vi "tic tac toe.vi"() -> ()   [LabVIEW 2017]
uses:
  <vilib>/event_ctls.llb/eventvkey.ctl
  <vilib>/DAQmx/write.llb/DAQmx Write (Digital Bool 1Line 1Point).vi
  <vilib>/DAQmx/read.llb/DAQmx Read (Counter U32 1Chan 1Samp).vi
  <vilib>/DAQmx/create/channels.llb/DAQmx Create Channel (CO-Pulse Generation-Frequency).vi
  <vilib>/DAQmx/configure/timing.llb/DAQmx Timing (Implicit).vi
  <vilib>/DAQmx/create/channels.llb/DAQmx Create Channel (CI-Count Edges).vi
  <vilib>/DAQmx/create/channels.llb/DAQmx Create Channel (DO-Digital Output).vi
  <vilib>/DAQmx/miscellaneous.llb/DAQmx Fill In Error Info.vi
  <resource>/objmgr/daqmx.rc
  <vilib>/Analysis/NI_AALBase.lvlib
panel:
  in  "btn pause":bool
  out "Станд. отклонение O":dbl format="%0.2f"
  out "Станд. отклонение X":dbl format="%0.2f"
  out "Мат. ождание O":dbl
  out "Мат. ождание X":dbl
  out "Гистограмма ходов O":T1(graph)
  out "Гистограмма ходов X":T1(graph)
  out "ВРЕМЯ ПОСЛЕДНЕГО ХОДА (сек.)":dbl
  out "Массив времён O":dbl[](array[numeric])
  out "Массив времён X":dbl[](array[numeric])
  out "Результат":string
  in  "btn new game":bool
  out "Boolean":bool
  in  "Игровое поле":i32[][](array[ring]) items=["", "X", "0"]
  out "ХОД":string
  in  "btn stop":bool
  # "\"Крестики-нолики 15x15\""
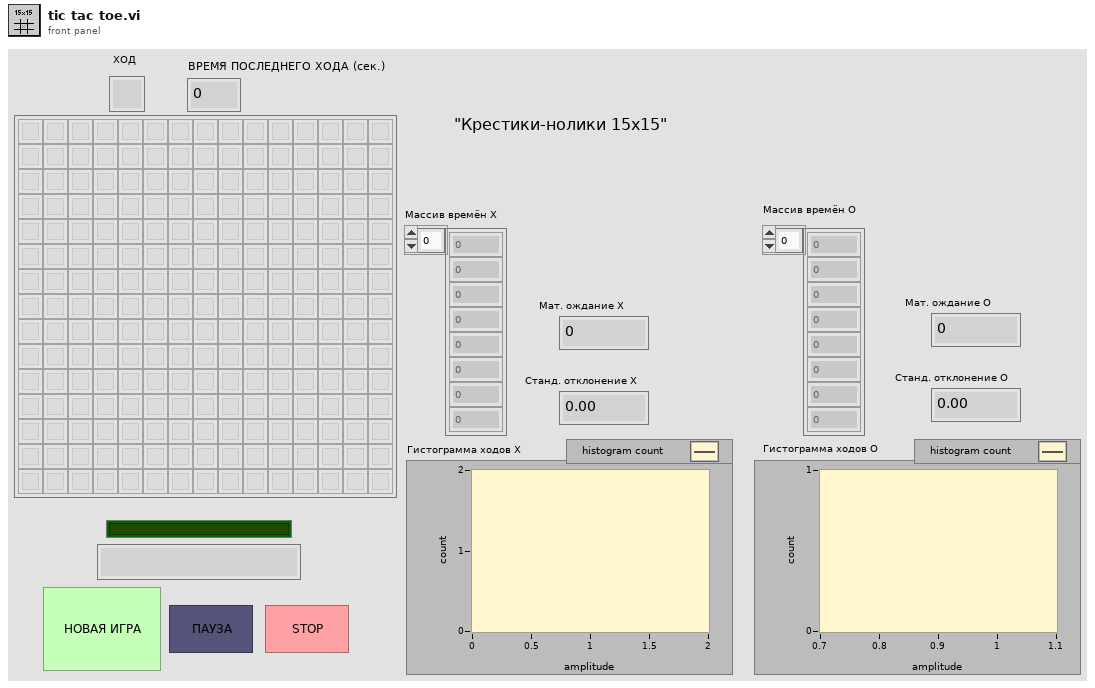
[diagram p1: front panel]
types:
  T1 = cluster{"X Values":dbl[], "Histogram: h(x)":i32[]}
  T2 = enum8{"Enabled", "Disabled", "Disabled and Grayed Out"}
  T3 = typedef "eventvkey.ctl" = enum16{"ASCII", "Enter", "Return", "Shift", "Ctrl", "Alt", "Cmd", "Opt", "Caps", "NumLock", "Clear", "Break", "Up", "Down", "Left", "Right", "Insert", "Delete", "Home", "End", "PageUp", "PageDown", "Escape", "Help", "Pause", "ScrollLock", "F1", "F2", "F3", "F4", "F5", "F6", "F7", "F8", "F9", "F10", "F11", "F12", "F13", "F14", "F15", "F16", "F17", "F18", "F19", "F20", "F21", "F22", "F23", "F24", "Play", "VolumeUp", "VolumeDown", "Mute", "Two Byte Char"}
  T4 = typedef "LVPoint32TypeDef.ctl" = cluster{"Horizontal":i32, "Vertical":i32}
  T5 = typedef "LVPositionTypeDef.ctl" = cluster{"Left":i32, "Top":i32}
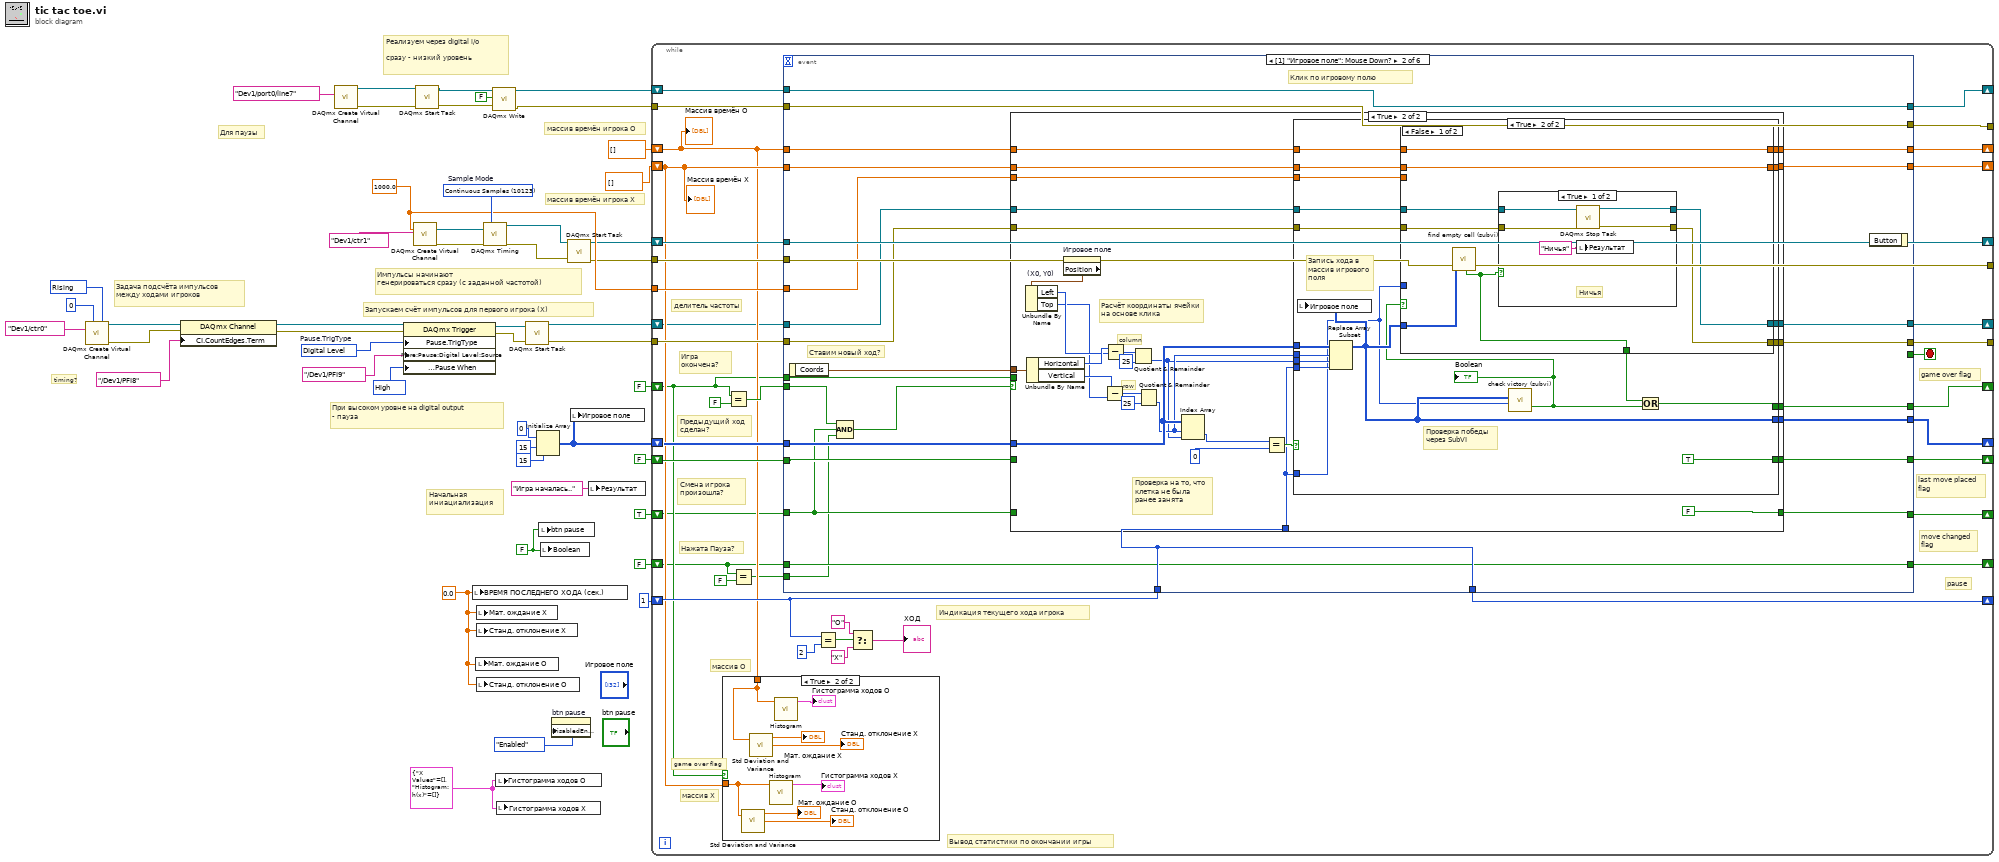
[diagram p0: block diagram]
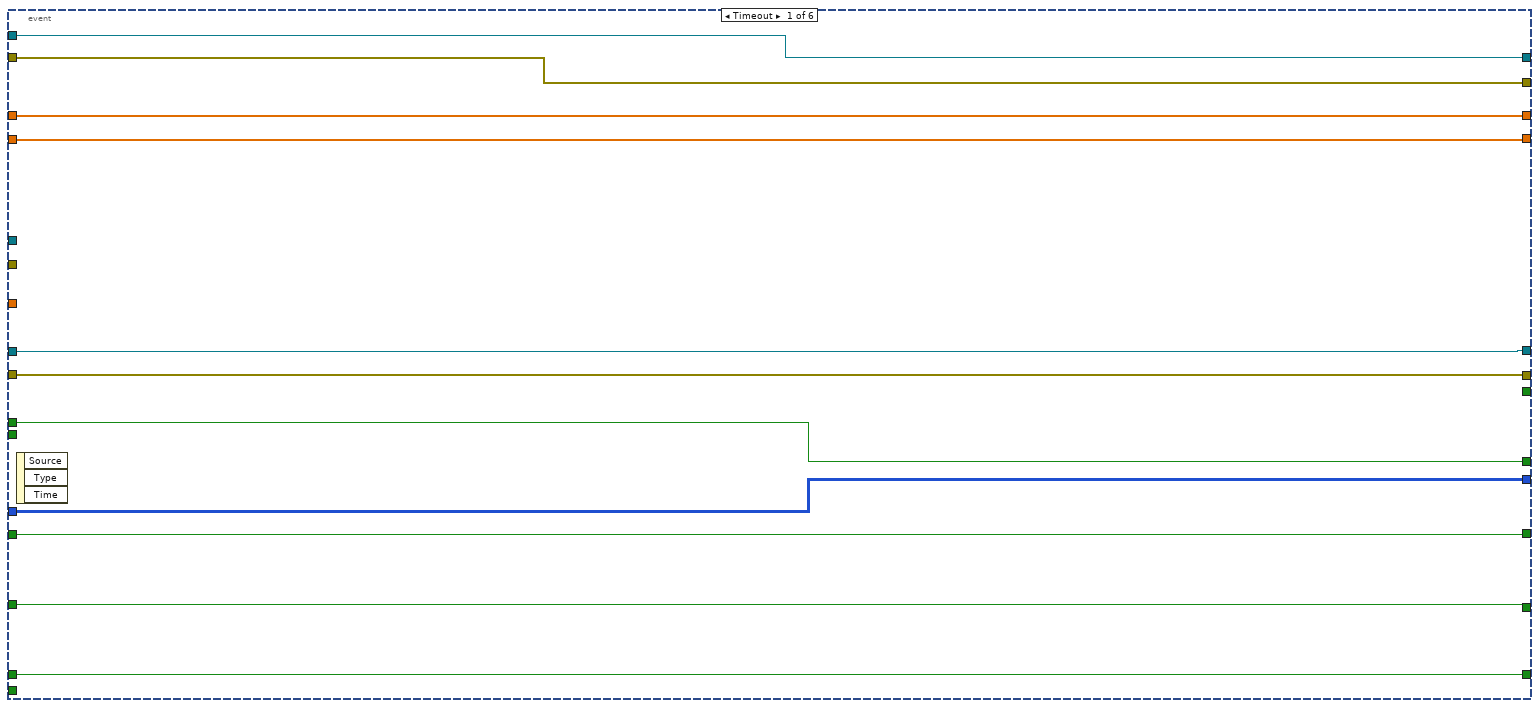
[diagram p3: hidden frame]
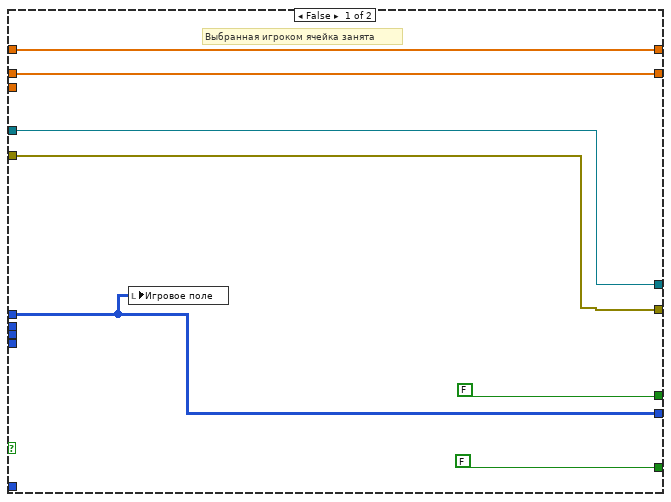
[diagram p5: hidden frame]
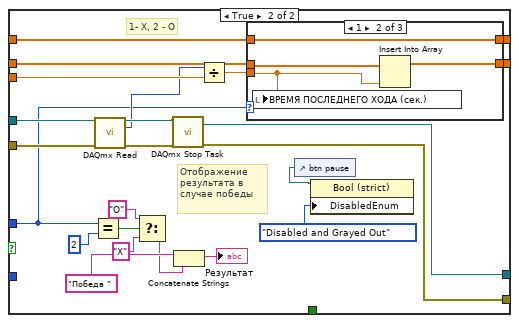
[diagram p7: hidden frame]
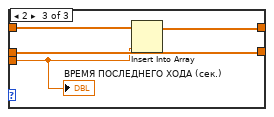
[diagram p9: hidden frame]
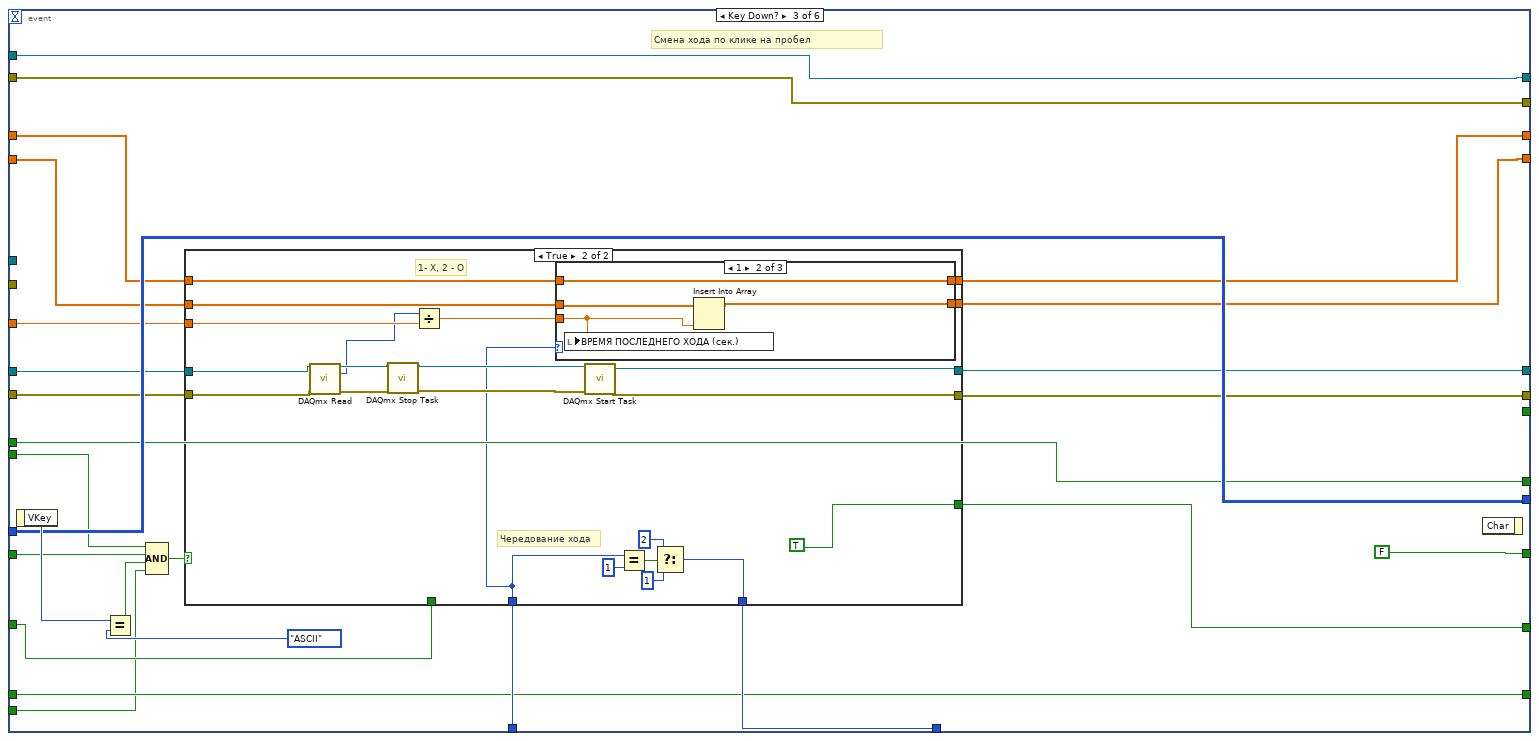
[diagram p10: hidden frame]
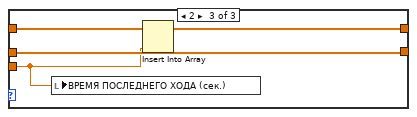
[diagram p13: hidden frame]
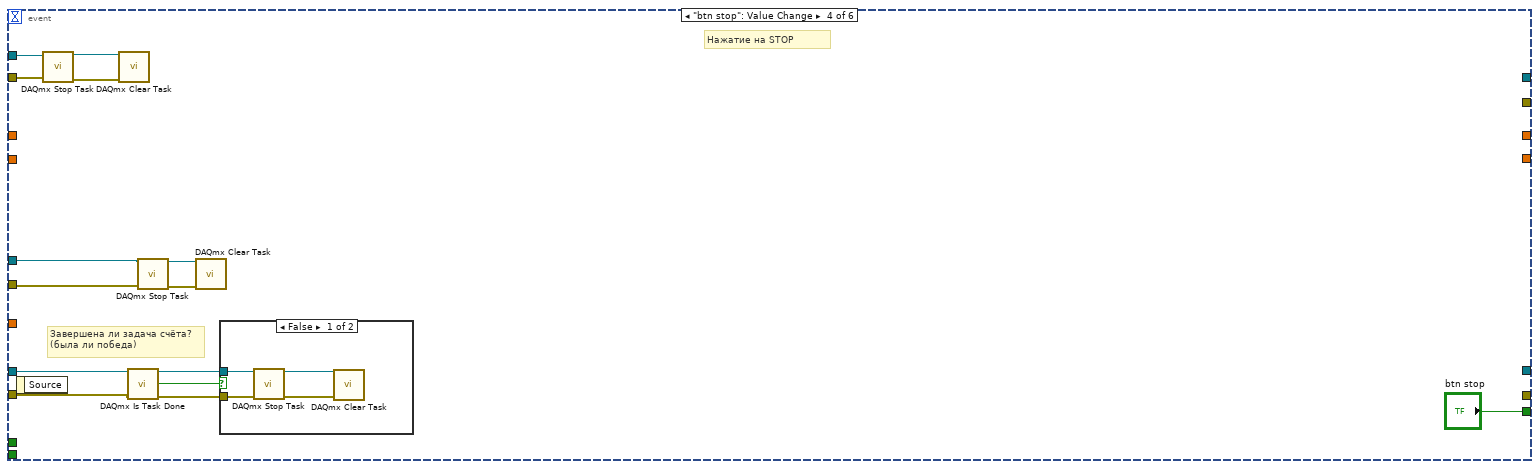
[diagram p14: hidden frame]
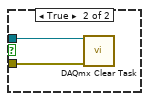
[diagram p15: hidden frame]
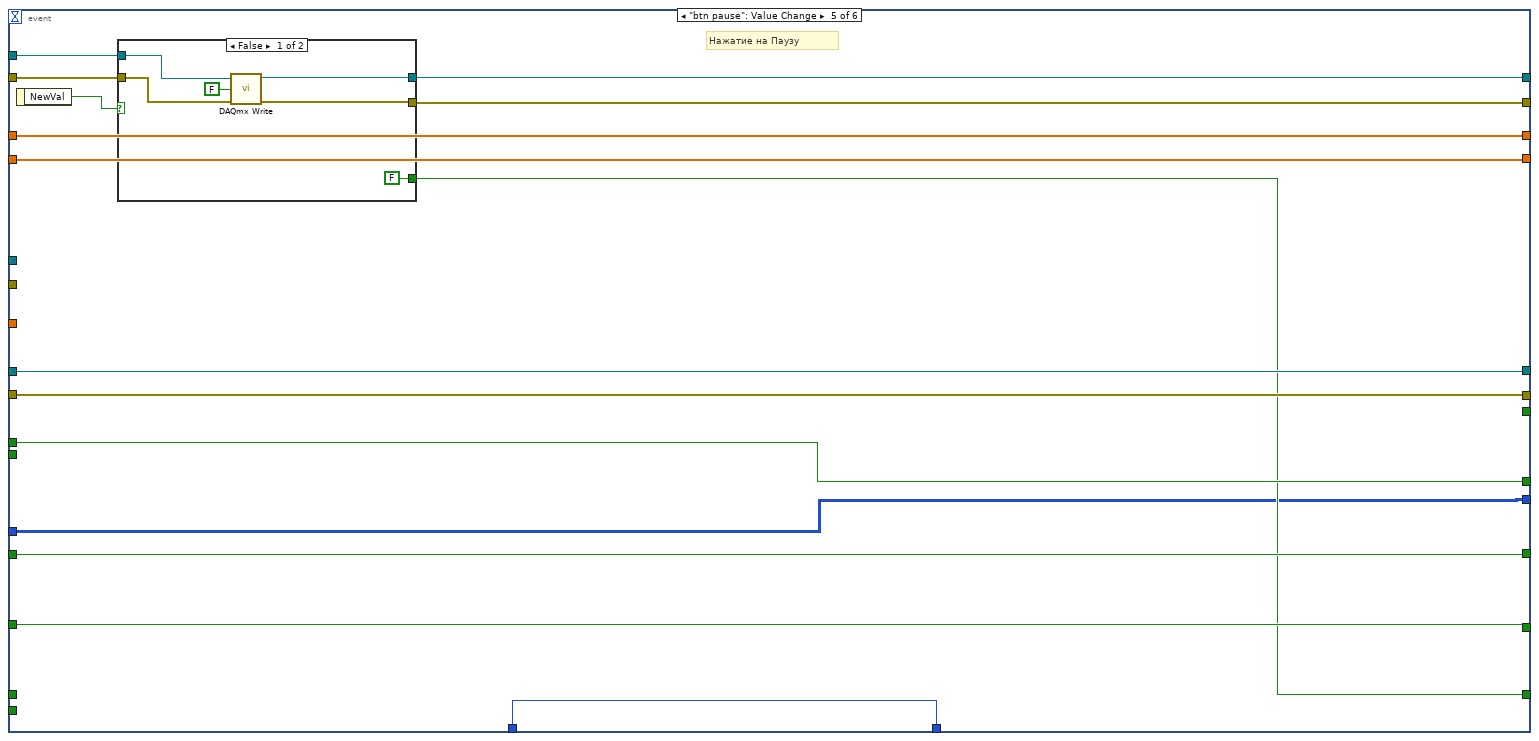
[diagram p16: hidden frame]
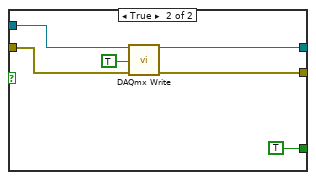
[diagram p17: hidden frame]
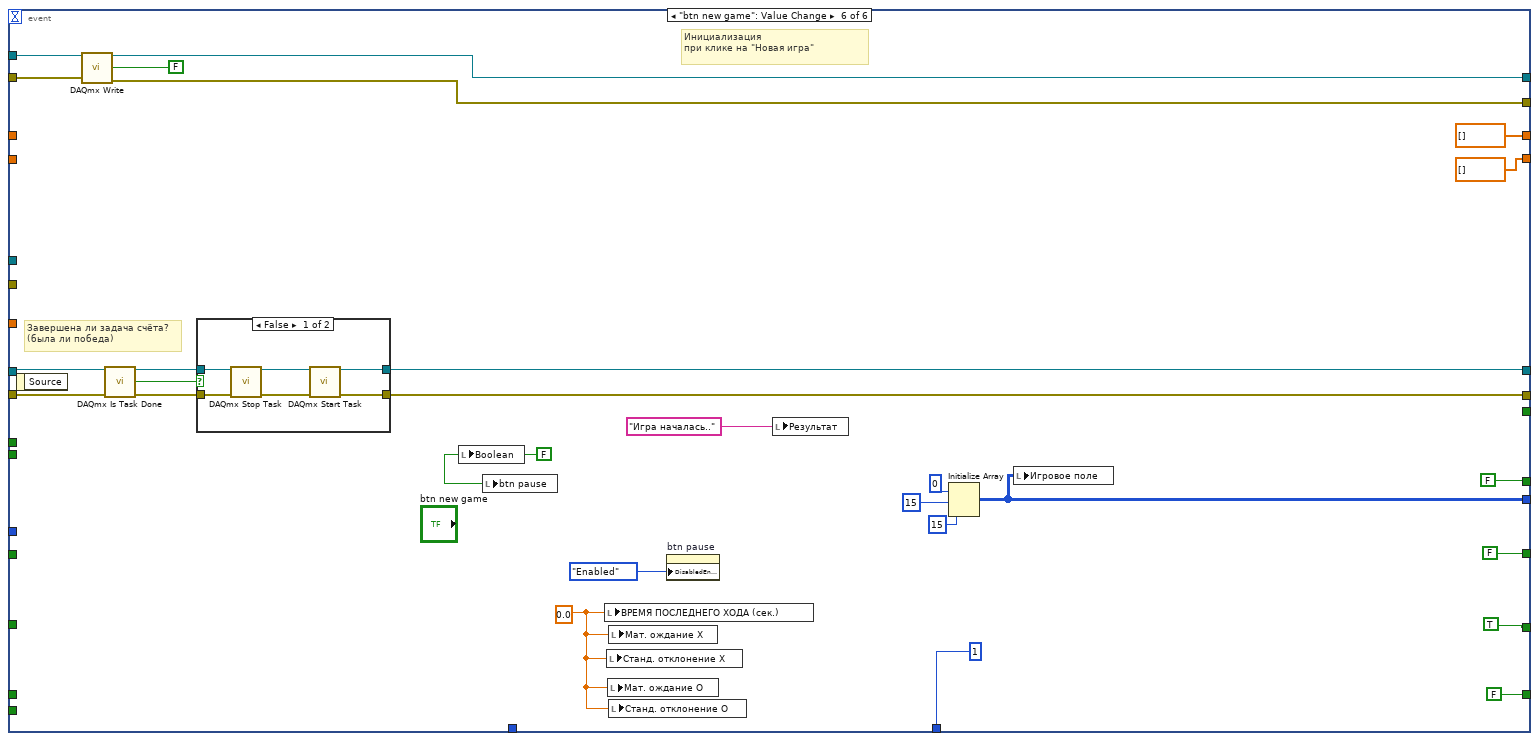
[diagram p18: hidden frame]
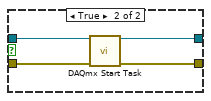
[diagram p19: hidden frame]
diagram:
  w1 = T1 {"X Values"=[], "Histogram: h(x)"=[]} ("Гистограмма ходов O")
  w2 = 0.0 ("Время последнего хода")
  w13 = 10192 items=["High"=10192, "Low"=10214] ("Pause When")
  w15 = 10152 items=["Analog Level"=10101, "Analog Window"=10103, "Digital Level"=10152, "Digital Pattern"=10398, "None"=10230]  # Pause.TrigType
  w32 = 10280 items=["Rising"=10280, "Falling"=10171] ("edge")
  w39 = 10123 items=["Finite Samples"=10178, "Continuous Samples"=10123, "Hardware Timed Single Point"=12522]  # Sample Mode
  w28 = 1000.0 ("frequency")
  w6 = FALSE
  # "При высоком уровне на digital output\n- пауза"
  # "Реализуем через digital i/o\n\nсразу - низкий уровень"
  # "Для паузы"
  # "массив времён игрока O"
  # "массив времён игрока X"
  # "Запускаем счёт импульсов для первого игрока (X)"
  # "Задача подсчёта импульсов\nмежду ходами игроков"
  # "timing?"
  # "Импульсы начинают\nгенерироваться сразу (с заданной частотой)"
  # "Начальная иниациализация"
  n1 = call-poly <vilib>:"DAQmx Create Virtual Channel.vi"("initial count"=u32 0, "edge"=w32, "counter"=tag "Dev1/ctr0") -> ("task out"=w30:refnum<k21>, "error out"=w29:errorcluster)  [unwired: 11 in]
  n2 = property class="DAQmx Channel"(reference=w30, error in=w29, "CI.CountEdges.Term"=tag "/Dev1/PFI8" ("CI.Period.Term")) -> (reference out=w10:refnum<k21>, error out=w9:errorcluster)
  n3 = call-poly <vilib>:"DAQmx Create Virtual Channel.vi"("lines"=tag "Dev1/port0/line7") -> ("task out"=w20:refnum<k21>, "error out"=w19:errorcluster)  [unwired: 13 in]
  n4 = property class="DAQmx Trigger"(reference=w10, error in=w9, "Pause.TrigType"=w15, "More:Pause:Digital Level:Source"=tag "/Dev1/PFI9" ("Pause Trigger Source"), "More:Pause:Digital Level:Pause When"=w13) -> (reference out=w12:refnum<k21>, error out=w11:errorcluster)
  n5 = call-poly <vilib>:"DAQmx Create Virtual Channel.vi"("frequency"=w28, "counter"=tag "Dev1/ctr1") -> ("task out"=w37:refnum<k21>, "error out"=w38:errorcluster)  [unwired: 12 in]
  n6 = call <vilib>:"DAQmx Start Task.vi"("task/channels in"=w20, "error in"=w19) -> ("task out"=w17:refnum<k21>, "error out"=w16:errorcluster)  [unwired: 12 in]
  n7 = local write "ВРЕМЯ ПОСЛЕДНЕГО ХОДА (сек.)"(w2) -> ()
  n8 = local write "Мат. ождание O"(w2) -> ()
  n9 = local write "Мат. ождание X"(w2) -> ()
  n10 = local write "Станд. отклонение X"(w2) -> ()
  n11 = local write "Станд. отклонение O"(w2) -> ()
  n12 = call-poly <vilib>:"DAQmx Timing.vi"("task/channels in"=w37, "sample mode"=w39, "error in"=w38) -> ("task out"=w36:refnum<k21>, "error out"=w35:errorcluster)  [unwired: 11 in]
  n13 = call-poly <vilib>:"DAQmx Write.vi"("task/channels in"=w17, "data"=FALSE, "error in"=w16) -> ("task out"=w8:refnum<k21>, "error out"=w7:errorcluster)  [unwired: 10 in, 1 out]
  n14 = local write "Гистограмма ходов O"(w1) -> ()
  n15 = local write "Гистограмма ходов X"(w1) -> ()
  n16 = call <vilib>:"DAQmx Start Task.vi"("task/channels in"=w12, "error in"=w11) -> ("task out"=w27:refnum<k21>, "error out"=w26:errorcluster)  [unwired: 12 in]
  n17 = Initialize Array(0 ("dimension size"), 15 ("dimension size"), 15 ("dimension size")) -> (w42:i32[][])
  n18 = local write "btn pause"(w6) -> ()
  n19 = local write "Boolean"(w6) -> ()
  n20 = property on="btn pause" class="Bool (strict)"("DisabledEnum"=T2."Enabled" ("Disabled")) -> ()  [unwired: 2 in, 2 out]
  n21 = call <vilib>:"DAQmx Start Task.vi"("task/channels in"=w36, "error in"=w35) -> ("task out"=w25:refnum<k21>, "error out"=w24:errorcluster)  [unwired: 12 in]
  n22 = local write "Игровое поле"(w42) -> ()
  n23 = local write "Результат"("Игра началась.." ("Результат")) -> ()
  n24 = while {
    shift-right: [w78] -> _
    shift-left: w42 -> [w79]
    shift-right: [w75] -> _
    shift-left: 1 ("f") -> [w76]
    shift-right: [w77] -> _
    shift-left: FALSE ("Победа") -> [w55]
    shift-right: [w74] -> _
    shift-left: FALSE -> [w73]
    shift-right: [w72] -> _
    shift-left: TRUE -> [w49]
    shift-right: [w69] -> _
    shift-left: w27 -> [w50]
    tunnel: w26 -> [w68]
    tunnel: w28 -> [w62]
    shift-right: [w67] -> _
    shift-left: w25 -> [w67]
    tunnel: w24 -> [w66]
    tunnel: [w66] -> _
    tunnel: [w65] -> _
    shift-right: [w64] -> _
    shift-left: dbl[] [] -> [w61]
    shift-right: [w63] -> _
    shift-left: dbl[] [] -> [w60]
    tunnel: w7 -> [w59]
    tunnel: [w58] -> _
    shift-right: [w56] -> _
    shift-left: w8 -> [w57]
    shift-right: [w54] -> _
    shift-left: FALSE -> [w52]
    stop <- w80 stop-if-true
    # "Нажата Пауза?"
    # "pause"
    # "делитель частоты"
    # "массив O"
    # "массив X"
    # "Вывод статистики по окончании игры"
    # "game over flag"
    # "Предыдущий ход сделан?"
    # "Смена игрока произошла?"
    # "Игра окончена?"
    # "move changed flag"
    # "last move placed\nflag"
    # "Индикация текущего хода игрока"
    # "game over flag"
    n25 = case shown="True" w55 {
      tunnel: w61 -> [_ w91]
      tunnel: w60 -> [_ w89]
      frame False {
      }
      frame True {
        n26 = call <vilib>:"Std Deviation and Variance.vi"("X"=w91) -> ("mean"=→"Мат. ождание O":dbl, "standard deviation"=→"Станд. отклонение O":dbl)  [unwired: 1 in, 1 out]
        n27 = call <vilib>:"Std Deviation and Variance.vi"("X"=w89) -> ("mean"=→"Мат. ождание X":dbl, "standard deviation"=→"Станд. отклонение X":dbl)  [unwired: 1 in, 1 out]
        n28 = call <vilib>:"Histogram.vi"("X"=w91) -> ("Histogram Graph"=→"Гистограмма ходов X":T1)  [unwired: 7 in, 3 out]
        n29 = call <vilib>:"Histogram.vi"("X"=w89) -> ("Histogram Graph"=→"Гистограмма ходов O":T1)  [unwired: 7 in, 3 out]
      }
    }
    n30 = Equal?(x=w55, y=FALSE) -> (x = y?=w70:bool)
    n31 = Equal?(x=w52, y=FALSE) -> (x = y?=w51:bool)
    n32 = event shown="[1] \"Игровое поле\": Mouse Down?" {
      selector: _ -> [_ _ _ _ _ _]
      dyn-events: _ -> [_ _ _ _ _ _]
      timeout: _ -> [_ _ _ _ _ _]
      tunnel: w79 -> [w94 w128 w263 _ w329 _]
      tunnel: w76 -> [_ w124 w266 _ w326 _]
      tunnel: [_ _ _ "btn stop" _ _] -> w80
      tunnel: [w94 w126 w263 _ w329 w376] -> w78
      tunnel: [w98 w127 w251 _ w333 FALSE] -> w77
      tunnel: w70 -> [_ w108 w246 _ _ _]
      tunnel: [_ w124 w265 _ w326 1] -> w75
      tunnel: [w102 w125 FALSE _ w335 FALSE] -> w74
      tunnel: w73 -> [w102 w122 w245 _ w335 _]
      tunnel: [w99 w123 w262 _ w334 TRUE] -> w72
      tunnel: w49 -> [w99 w107 w248 _ w334 _]
      tunnel: w50 -> [w104 w120 w260 w312 w332 w371]
      tunnel: [w104 w119 w259 _ w332 w366] -> w69
      tunnel: w68 -> [w103 w121 w258 w311 w331 w370]
      tunnel: [w103 w118 w257 _ w331 w365] -> w65
      tunnel: w62 -> [_ w112 w256 _ _ _]
      tunnel: w67 -> [_ _ _ w314 _ _]
      tunnel: w66 -> [_ _ _ w313 _ _]
      tunnel: [w100 w117 w252 _ w327 dbl[] []] -> w64
      tunnel: w61 -> [w100 w116 w254 _ w327 _]
      tunnel: [w101 w115 w253 _ w328 dbl[] []] -> w63
      tunnel: w60 -> [w101 w114 w255 _ w328 _]
      tunnel: w57 -> [w97 w111 w250 w309 w339 w360]
      tunnel: w59 -> [w96 w110 w249 w308 w338 w359]
      tunnel: [w97 w111 w250 _ w337 w357] -> w56
      tunnel: [w96 w110 w249 _ w336 w356] -> w58
      tunnel: w55 -> [w98 w113 w251 _ w333 _]
      tunnel: [w95 w109 w247 _ w330 FALSE] -> w54
      tunnel: w52 -> [w95 w109 w247 _ _ _]
      tunnel: w51 -> [_ w106 w243 _ _ _]
      event Timeout {
        n33 = event-data() -> ()  [unwired: 1 in, 3 out]
      }
      event "Игровое поле": Mouse Down? {
        # "Клик по игровому полю"
        # "Ставим новый ход?"
        n34 = event-data() -> ("Coords"=w129:T4)  [unwired: 1 in]
        n35 = Compound Arithmetic op=AND(w108, w107, w106) -> (w105:bool)
        n36 = case shown="True" w105 {
          tunnel: w124 -> [_ w149]
          tunnel: w129 -> [_ w167]
          tunnel: w128 -> [w137 w157]
          tunnel: [w130 w151] -> w127
          tunnel: [w137 w150] -> w126
          tunnel: [w135 w148] -> w125
          tunnel: [w136 FALSE] -> w123
          tunnel: w107 -> [w136 _]
          tunnel: w122 -> [w135 _]
          tunnel: w112 -> [_ w146]
          tunnel: w120 -> [w134 w145]
          tunnel: w121 -> [w133 w144]
          tunnel: [w134 w143] -> w119
          tunnel: [w133 w142] -> w118
          tunnel: [w132 w141] -> w117
          tunnel: w116 -> [w132 w140]
          tunnel: [w131 w139] -> w115
          tunnel: w114 -> [w131 w138]
          tunnel: w113 -> [w130 _]
          frame False {
          }
          frame True {
            # "Расчёт координаты ячейки\nна основе клика"
            # "Проверка на то, что клетка не была ранее занята"
            # "row"
            # "column"
            n37 = Unbundle By Name(w167) -> ("Horizontal"=w165:i32, "Vertical"=w159:i32)
            n38 = property on="Игровое поле" class="Arr (strict)"() -> ("Position"=w166:T5)  [unwired: 2 in, 2 out]
            n39 = Unbundle By Name "(X0, Y0)"(w166) -> ("Left"=w164:i32, "Top"=w158:i32)
            n40 = Subtract(x=w159, y=w158) -> (x-y=w161:i32)
            n41 = Subtract(x=w165, y=w164) -> (x-y=w163:i32)
            n42 = Quotient & Remainder(x=w163, y=25) -> (floor(x/y)=w155:i32)  [unwired: 1 out]
            n43 = Quotient & Remainder(x=w161, y=25) -> (floor(x/y)=w156:i32)  [unwired: 1 out]
            n44 = Index Array(array=w157, index (row)=w156, index (col)=w155) -> (element=w153:i32)
            n45 = Equal?(x=w153, y=0 ("dimension size")) -> (x = y?=w152:bool)
            n46 = case shown="True" w152 {
              tunnel: w149 -> [_ w184]
              tunnel: w149 -> [_ w193]
              tunnel: [FALSE w186] -> w151
              tunnel: w157 -> [w173 w192]
              tunnel: w156 -> [_ w191]
              tunnel: w155 -> [_ w190]
              tunnel: [w173 w189] -> w150
              tunnel: [FALSE TRUE] -> w148
              tunnel: w146 -> [_ w183]
              tunnel: w145 -> [w171 w182]
              tunnel: w144 -> [w170 w181]
              tunnel: [w171 w180] -> w143
              tunnel: [w170 w179] -> w142
              tunnel: [w169 w178] -> w141
              tunnel: w140 -> [w169 w177]
              tunnel: [w168 w176] -> w139
              tunnel: w138 -> [w168 w175]
              frame False {
                # "Выбранная игроком ячейка занята"
                n47 = local write "Игровое поле"(w173) -> ()
              }
              frame True {
                # "Запись хода в массив игрового поля"
                # "Проверка победы\nчерез SubVI"
                n48 = Replace Array Subset(array=w192, new element=w193, index (row)=w191, index (col)=w190) -> (w189:i32[][])
                n49 = local write "Игровое поле"(w189) -> ()
                n50 = call "check victory (subvi).vi"("Игрок"=w184, "Игровое поле"=w189) -> ("Победа"=w188:bool)  [unwired: 9 in]
                "Boolean" <- w188
                n51 = case shown="False" w188 {
                  tunnel: w184 -> [_ w213]
                  tunnel: w189 -> [w201 _]
                  tunnel: [w200 _] -> w187
                  tunnel: w183 -> [_ w224]
                  tunnel: w182 -> [w195 w223]
                  tunnel: w181 -> [w197 w222]
                  tunnel: [w194 w221] -> w180
                  tunnel: [w196 w220] -> w179
                  tunnel: [w199 w219] -> w178
                  tunnel: w177 -> [w199 w218]
                  tunnel: [w198 w212] -> w176
                  tunnel: w175 -> [w198 w211]
                  frame False {
                    n52 = call "find empty cell (subvi).vi"("Array"=w201) -> ("Ничья"=w200:bool)  [unwired: 10 in]
                    n53 = case shown="True" w200 {
                      tunnel: w197 -> [w204 w208]
                      tunnel: [w203 w208] -> w196
                      tunnel: w195 -> [w205 w207]
                      tunnel: [w202 w207] -> w194
                      frame True {
                        # "Ничья"
                        n54 = call <vilib>:"DAQmx Stop Task.vi"("task/channels in"=w205, "error in"=w204) -> ("task out"=w202:refnum<k21>, "error out"=w203:errorcluster)  [unwired: 12 in]
                        n55 = local write "Результат"("Ничья") -> ()
                      }
                      frame False {
                      }
                    }
                  }
                  frame True {
                    # "1- X, 2 - O"
                    # "Отображение результата в случае победы"
                    n56 = Equal?(x=w213, y=2) -> (x = y?=w230:bool)
                    n57 = call-poly <vilib>:"DAQmx Read.vi"("task/channels in"=w223, "error in"=w222) -> ("task out"=w216:refnum<k21>, "data"=w215:u32, "error out"=w217:errorcluster)  [unwired: 11 in]
                    n58 = Select(t="O", s=w230, f="X") -> (s? t:f=w226:string)
                    n59 = call <vilib>:"DAQmx Stop Task.vi"("task/channels in"=w216, "error in"=w217) -> ("task out"=w221:refnum<k21>, "error out"=w220:errorcluster)  [unwired: 12 in]
                    n60 = Concatenate Strings("Победа ", w226) -> (→"Результат":string)
                    n61 = Divide(x=w215, y=w224) -> (x/y=w214:dbl)
                    n62 = case shown="1" w213 {
                      tunnel: [w232 w237 w241] -> w219
                      tunnel: w218 -> [w232 w234 w241]
                      tunnel: w214 -> [_ w235 w238]
                      tunnel: [w233 w236 w240] -> w212
                      tunnel: w211 -> [w233 w236 w239]
                      frame 0, Default {
                      }
                      frame 1 {
                        n63 = local write "ВРЕМЯ ПОСЛЕДНЕГО ХОДА (сек.)"(w235) -> ()
                        n64 = Insert Into Array(array=w234, new element=w235) -> (w237:dbl[])  [unwired: 1 in]
                      }
                      frame 2 {
                        n65 = Insert Into Array(array=w239, new element=w238) -> (w240:dbl[])  [unwired: 1 in]
                        "ВРЕМЯ ПОСЛЕДНЕГО ХОДА (сек.)" <- w238
                      }
                    }
                    n66 = control-ref of="btn pause"() -> (w209:refnum<vi>)
                    n67 = property class="Bool (strict)"(reference=w209, "DisabledEnum"=T2."Disabled and Grayed Out" ("Disabled")) -> ()  [unwired: 1 in, 2 out]
                  }
                }
                n68 = Or(x=w187, y=w188) -> (x .or. y?=w186:bool)
              }
            }
          }
        }
        n69 = event-data() -> ()  [unwired: 2 in, 1 out]
      }
      event Key Down? {
        # "Смена хода по клике на пробел"
        n70 = event-data() -> ("VKey"=w267:T3)  [unwired: 1 in]
        n71 = Equal?(x=w267, y=eventvkey."ASCII") -> (x = y?=w244:bool)
        n72 = Compound Arithmetic op=AND(w246, w245, w244, w243) -> (w242:bool)
        n73 = case shown="True" w242 {
          tunnel: w266 -> [w273 w279]
          tunnel: [w273 w295] -> w265
          tunnel: [w268 TRUE] -> w262
          tunnel: w260 -> [w272 w284]
          tunnel: [w272 w289] -> w259
          tunnel: w258 -> [w271 w285]
          tunnel: [w271 w288] -> w257
          tunnel: w256 -> [_ w281]
          tunnel: w255 -> [w270 w278]
          tunnel: w254 -> [w269 w277]
          tunnel: [w270 w276] -> w253
          tunnel: [w269 w275] -> w252
          tunnel: w248 -> [w268 _]
          frame False {
          }
          frame True {
            # "1- X, 2 - O"
            # "Чередование хода"
            n74 = call-poly <vilib>:"DAQmx Read.vi"("task/channels in"=w284, "error in"=w285) -> ("task out"=w286:refnum<k21>, "data"=w280:u32, "error out"=w287:errorcluster)  [unwired: 11 in]
            n75 = call <vilib>:"DAQmx Stop Task.vi"("task/channels in"=w286, "error in"=w287) -> ("task out"=w282:refnum<k21>, "error out"=w283:errorcluster)  [unwired: 12 in]
            n76 = Divide(x=w280, y=w281) -> (x/y=w274:dbl)
            n77 = case shown="1" w279 {
              tunnel: [w296 w301 w305] -> w275
              tunnel: w277 -> [w296 w300 w305]
              tunnel: w274 -> [_ w298 w302]
              tunnel: [w297 w299 w304] -> w276
              tunnel: w278 -> [w297 w299 w303]
              frame 0, Default {
              }
              frame 1 {
                n78 = local write "ВРЕМЯ ПОСЛЕДНЕГО ХОДА (сек.)"(w298) -> ()
                n79 = Insert Into Array(array=w300, new element=w298) -> (w301:dbl[])  [unwired: 1 in]
              }
              frame 2 {
                n80 = local write "ВРЕМЯ ПОСЛЕДНЕГО ХОДА (сек.)"(w302) -> ()
                n81 = Insert Into Array(array=w303, new element=w302) -> (w304:dbl[])  [unwired: 1 in]
              }
            }
            n82 = call <vilib>:"DAQmx Start Task.vi"("task/channels in"=w282, "error in"=w283) -> ("task out"=w289:refnum<k21>, "error out"=w288:errorcluster)  [unwired: 12 in]
            n83 = Equal?(x=w279, y=1) -> (x = y?=w293:bool)
            n84 = Select(t=2, s=w293, f=1) -> (s? t:f=w295:i32)
          }
        }
        n85 = event-data() -> ()  [unwired: 2 in, 1 out]
      }
      event "btn stop": Value Change {
        # "Нажатие на STOP"
        # "Завершена ли задача счёта?\n(была ли победа)"
        n86 = event-data() -> ()  [unwired: 1 in, 1 out]
        n87 = call <vilib>:"DAQmx Stop Task.vi"("task/channels in"=w309, "error in"=w308) -> ("task out"=w306:refnum<k21>, "error out"=w307:errorcluster)  [unwired: 12 in]
        n88 = call <vilib>:"DAQmx Clear Task.vi"("task in"=w306, "error in"=w307) -> ()  [unwired: 13 in, 1 out]
        n89 = call <vilib>:"DAQmx Is Task Done.vi"("task/channels in"=w312, "error in"=w311) -> ("task out"=w317:refnum<k21>, "task done?"=w318:bool, "error out"=w316:errorcluster)  [unwired: 11 in]
        n90 = call <vilib>:"DAQmx Stop Task.vi"("task/channels in"=w314, "error in"=w313) -> ("task out"=w315:refnum<k21>, "error out"=w310:errorcluster)  [unwired: 12 in]
        n91 = call <vilib>:"DAQmx Clear Task.vi"("task in"=w315, "error in"=w310) -> ()  [unwired: 13 in, 1 out]
        n92 = case shown="False" w318 {
          tunnel: w317 -> [w323 w325]
          tunnel: w316 -> [w322 w324]
          frame False {
            n93 = call <vilib>:"DAQmx Stop Task.vi"("task/channels in"=w323, "error in"=w322) -> ("task out"=w321:refnum<k21>, "error out"=w320:errorcluster)  [unwired: 12 in]
            n94 = call <vilib>:"DAQmx Clear Task.vi"("task in"=w321, "error in"=w320) -> ()  [unwired: 13 in, 1 out]
          }
          frame True {
            n95 = call <vilib>:"DAQmx Clear Task.vi"("task in"=w325, "error in"=w324) -> ()  [unwired: 13 in, 1 out]
          }
        }
      }
      event "btn pause": Value Change {
        # "Нажатие на Паузу"
        n96 = event-data() -> ("NewVal"=w340:bool)  [unwired: 1 in]
        n97 = case shown="False" w340 {
          tunnel: w339 -> [w345 w351]
          tunnel: w338 -> [w342 w350]
          tunnel: [w344 w349] -> w337
          tunnel: [w343 w348] -> w336
          tunnel: [FALSE TRUE] -> w330
          frame False {
            n98 = call-poly <vilib>:"DAQmx Write.vi"("task/channels in"=w345, "data"=FALSE, "error in"=w342) -> ("task out"=w344:refnum<k21>, "error out"=w343:errorcluster)  [unwired: 10 in, 1 out]
          }
          frame True {
            n99 = call-poly <vilib>:"DAQmx Write.vi"("task/channels in"=w351, "data"=TRUE, "error in"=w350) -> ("task out"=w349:refnum<k21>, "error out"=w348:errorcluster)  [unwired: 10 in, 1 out]
          }
        }
      }
      event "btn new game": Value Change {
        w353 = 0.0 ("Время последнего хода")
        w361 = FALSE ("Boolean")
        # "Завершена ли задача счёта?\n(была ли победа)"
        # "Инициализация\nпри клике на \"Новая игра\""
        n100 = event-data() -> ()  [unwired: 1 in, 1 out]
        n101 = call-poly <vilib>:"DAQmx Write.vi"("task/channels in"=w360, "data"=FALSE, "error in"=w359) -> ("task out"=w357:refnum<k21>, "error out"=w356:errorcluster)  [unwired: 10 in, 1 out]
        n102 = call <vilib>:"DAQmx Is Task Done.vi"("task/channels in"=w371, "error in"=w370) -> ("task out"=w368:refnum<k21>, "task done?"=w369:bool, "error out"=w367:errorcluster)  [unwired: 11 in]
        n103 = case shown="False" w369 {
          tunnel: w368 -> [w385 w389]
          tunnel: w367 -> [w384 w388]
          tunnel: [w381 w387] -> w366
          tunnel: [w380 w386] -> w365
          frame False {
            n104 = call <vilib>:"DAQmx Stop Task.vi"("task/channels in"=w385, "error in"=w384) -> ("task out"=w383:refnum<k21>, "error out"=w382:errorcluster)  [unwired: 12 in]
            n105 = call <vilib>:"DAQmx Start Task.vi"("task/channels in"=w383, "error in"=w382) -> ("task out"=w381:refnum<k21>, "error out"=w380:errorcluster)  [unwired: 12 in]
          }
          frame True {
            n106 = call <vilib>:"DAQmx Start Task.vi"("task/channels in"=w389, "error in"=w388) -> ("task out"=w387:refnum<k21>, "error out"=w386:errorcluster)  [unwired: 12 in]
          }
        }
        n107 = local write "Boolean"(w361) -> ()
        n108 = local write "btn pause"(w361) -> ()
        n109 = local write "ВРЕМЯ ПОСЛЕДНЕГО ХОДА (сек.)"(w353) -> ()
        n110 = local write "Станд. отклонение X"(w353) -> ()
        n111 = local write "Мат. ождание O"(w353) -> ()
        n112 = local write "Мат. ождание X"(w353) -> ()
        n113 = local write "Станд. отклонение O"(w353) -> ()
        n114 = property on="btn pause" class="Bool (strict)"("DisabledEnum"=T2."Enabled" ("Disabled")) -> ()  [unwired: 2 in, 2 out]
        n115 = local write "Результат"("Игра началась.." ("Результат")) -> ()
        n116 = Initialize Array(0 ("dimension size"), 15 ("dimension size"), 15 ("dimension size")) -> (w376:i32[][])
        n117 = local write "Игровое поле"(w376) -> ()
      }
    }
    n118 = Equal?(x=w76, y=2) -> (x = y?=w85:bool)
    n119 = Select(t="O", s=w85, f="X") -> (s? t:f=→"ХОД":string)
    "Массив времён X" <- w61
    "Массив времён O" <- w60
  }
